vi "LiveAcquire20161118.vi"() -> ()   [LabVIEW 2015]
uses:
  <userlib>/atmcd64d.llb/AcquisitionMode_mode typedef.ctl
  NIDAQControls/StateGlobals.vi
  AcquisitionGlobals.vi
  NIDAQControls/NIDAQGlobals.vi
  LiveImage_Global.vi
panel:
  out "overflow?":bool
  out "deltat":u64
  out "arr":u64[](array[numeric])
  out "size(s) 2":i32
  out "size(s)":i32
  out "xpixels 2":i32
  out "ypixels 2":i32
  out "Acquire Time":dbl
  out "Wait Time":dbl
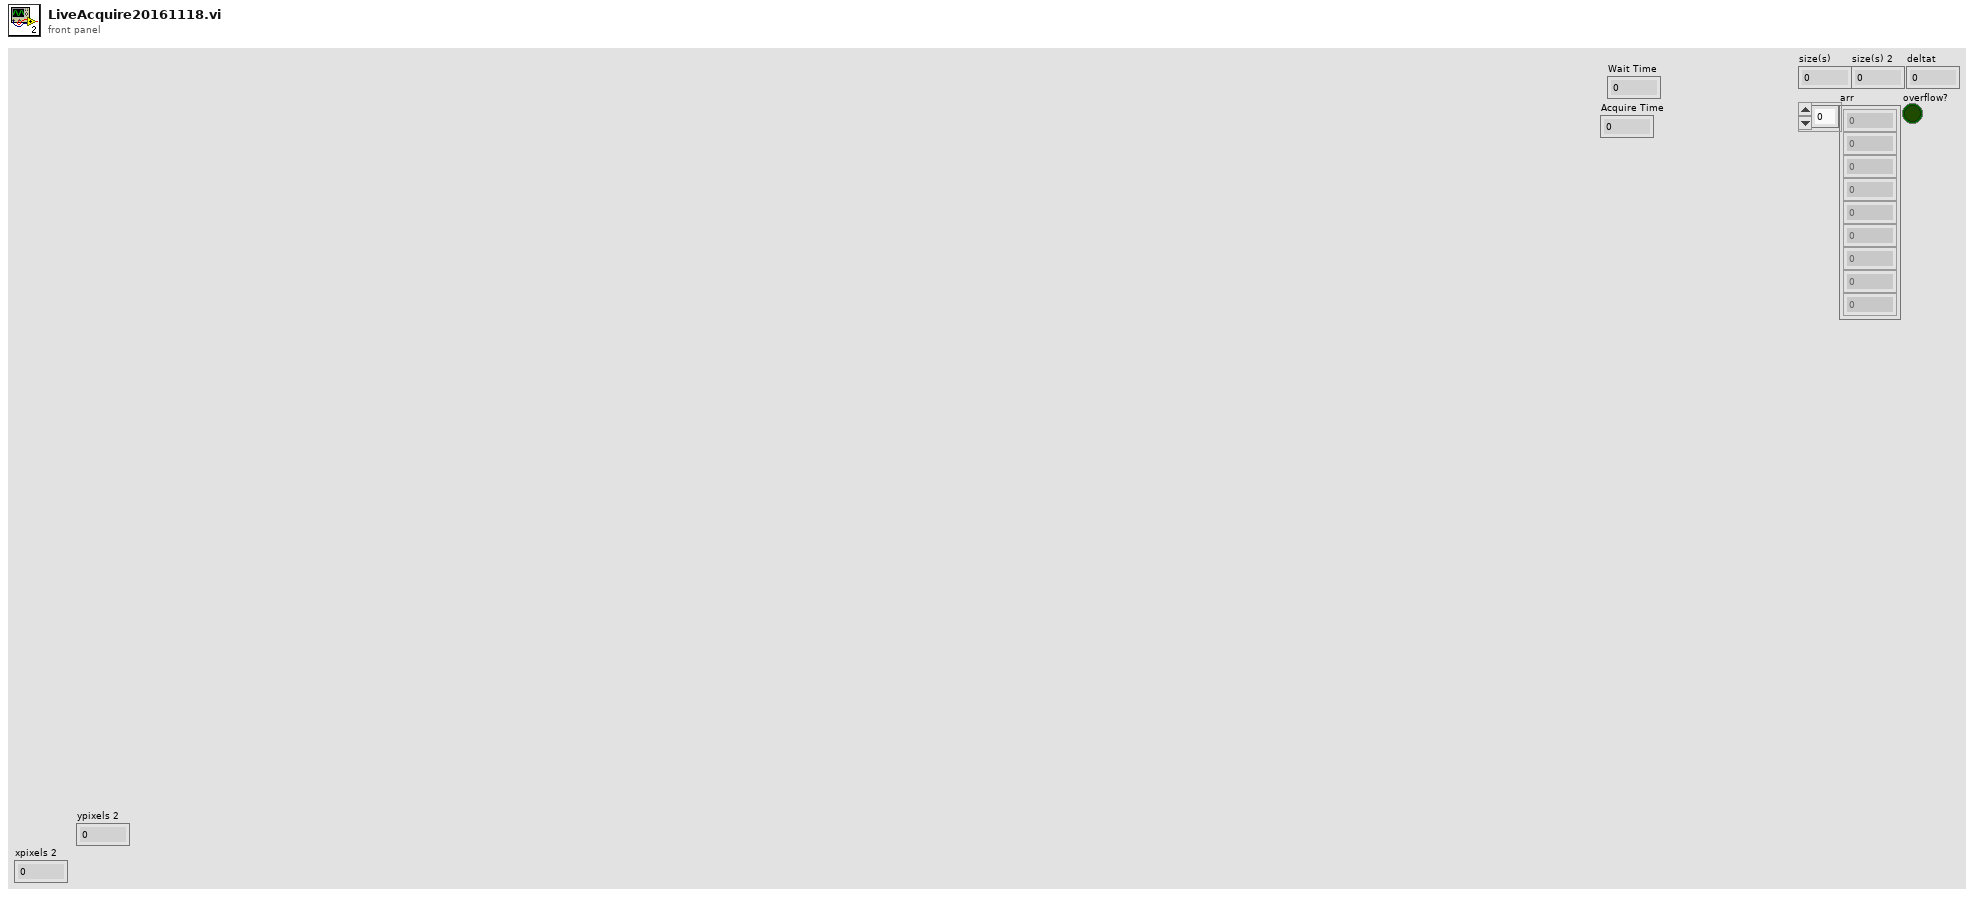
[diagram p1: front panel]
types:
  T1 = cluster{"Start or New Parameters?":bool, "Laser Mode":string, "Piezo Mode":string, "Begin Or End Acquisition":string, "Acquisition Time":dbl}
  T2 = enum16{"Create", "Lossy Enqueue", "Enqueue", "Dequeue", "Destroy"}
  T3 = typedef "AcquisitionMode_mode typedef.ctl" = enum16{"Reserved (0)", "Single Scan", "Accumulate", "Kinetics", "Fast Kinetics", "Run Till Abort", "Reserved (6)", "Reserved (7)", "Reserved (8)", "Time Delayed Integration"}
  T4 = typedef "Rendezvous RefNum" = refnum<k1>
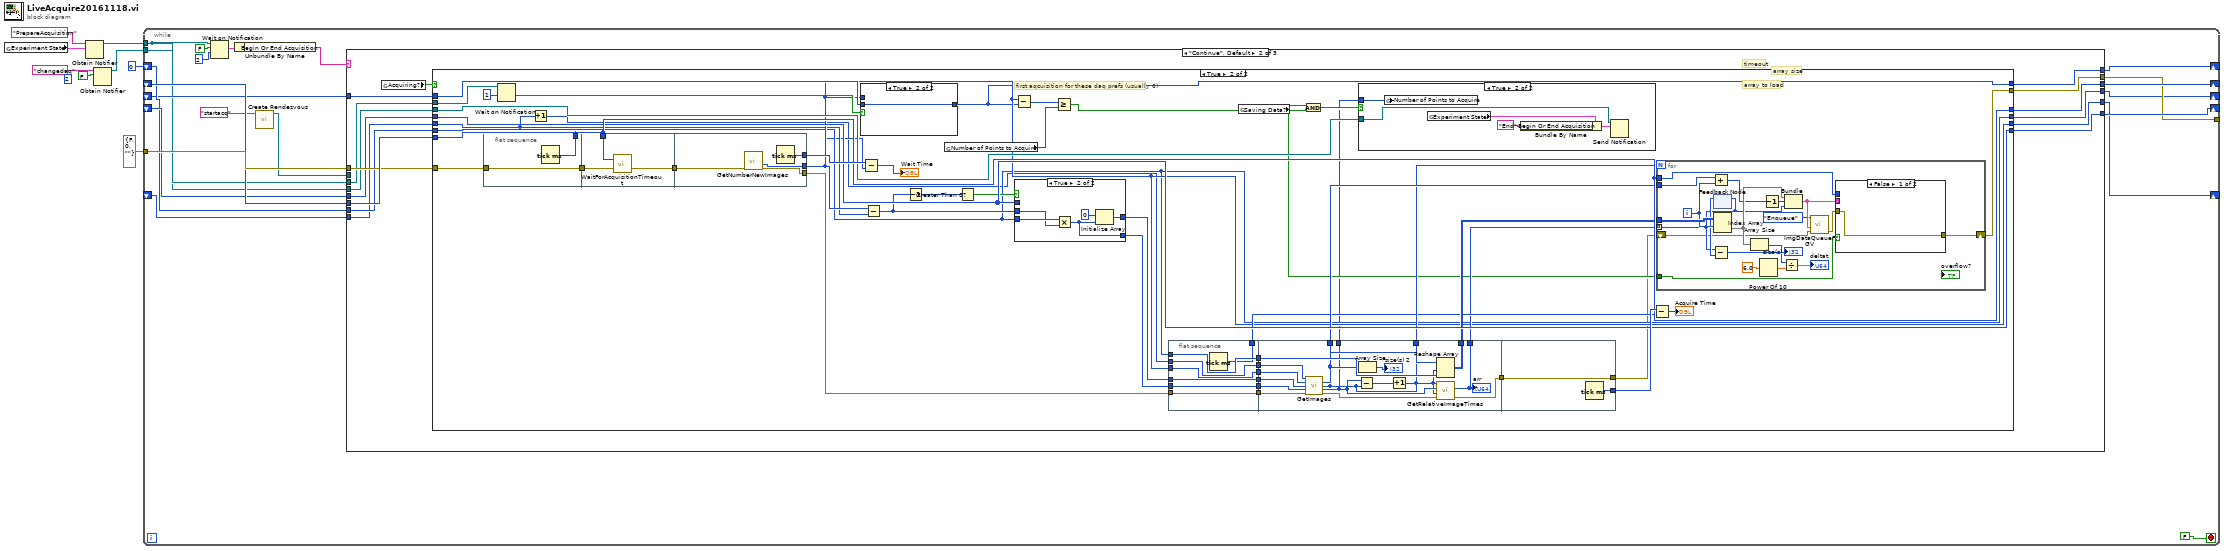
[diagram p0: block diagram]
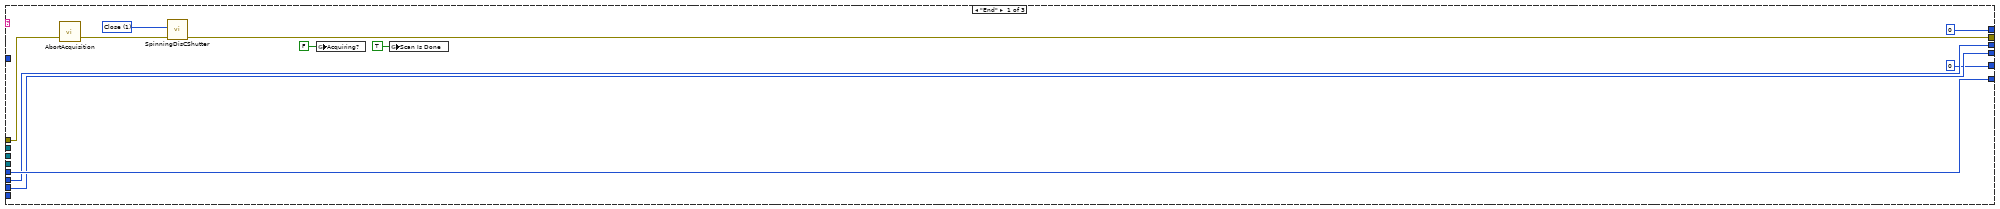
[diagram p2: hidden frame]
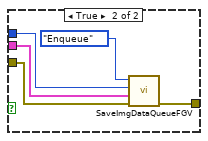
[diagram p4: hidden frame]
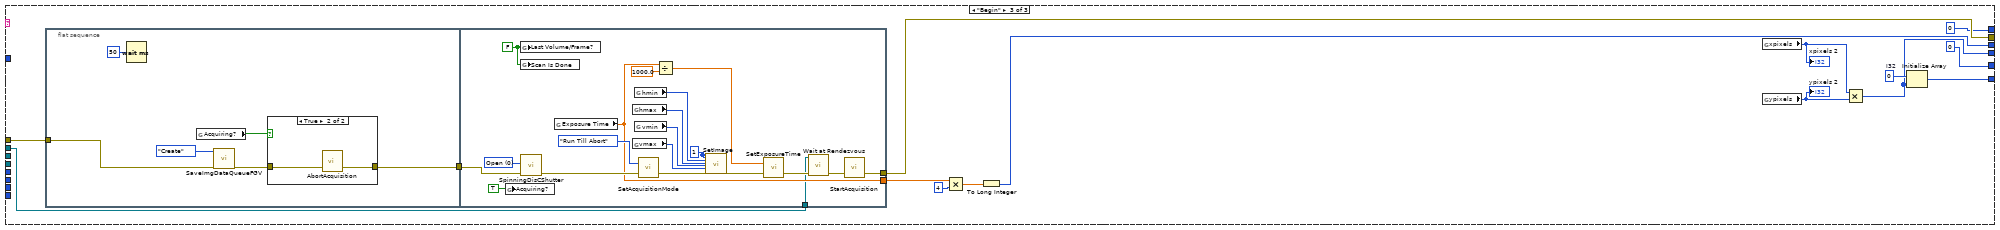
[diagram p8: hidden frame]
diagram:
  (unwired) 2 ("max queue size (-1, unlimited)")
  n1 = global read "StateGlobals.vi" "Experiment State"() -> (w1:T1)
  n2 = Obtain Notifier(name (unnamed)="PrepareAcquisition", notification data type=w1) -> (notifier out=w6:refnum<notifier>)  [unwired: 2 in, 2 out]
  n3 = Obtain Notifier(name (unnamed)="changedaq", notification data type=FALSE) -> (notifier out=w2:refnum<notifier>)  [unwired: 2 in, 2 out]
  n4 = while {
    tunnel: w6 -> [w12]
    shift-right: [w26] -> _
    shift-left: _ -> [w22]
    shift-right: [w25] -> _
    shift-left: _ -> [w21]
    shift-right: [w11] -> _
    shift-left: _ -> [w19]
    tunnel: errorcluster {"status"=FALSE, "code"=0, "source"=""} ("error out") -> [w24]
    tunnel: [w23] -> _
    shift-right: [w14] -> _
    shift-left: 0 -> [w15]
    tunnel: w2 -> [w13]
    shift-right: [w9] -> _
    shift-left: _ -> [w10]
    stop <- FALSE stop-if-true
    # "array size"
    # "timeout"
    # "array to load"
    n5 = Wait on Notification(notifier=w12, ignore previous (F)=FALSE, timeout in ms (-1)=2) -> (notification=w28:T1)  [unwired: 1 in, 3 out]
    n6 = Unbundle By Name(w28) -> ("Begin Or End Acquisition"=w27:string)
    n7 = call <vilib>:"Create Rendezvous.vi"("name (unnamed)"="startacq") -> ("rendezvous"=w17:T4)  [unwired: 4 in, 2 out]
    n8 = case shown="\"Continue\", Default" w27 {
      tunnel: [w33 w48 w191] -> w26
      tunnel: [w35 w49 w190] -> w25
      tunnel: [w34 w47 w189] -> w11
      tunnel: w24 -> [w36 w53 w188]
      tunnel: [w30 w50 w187] -> w23
      tunnel: w22 -> [w33 w54 _]
      tunnel: w21 -> [w35 w52 _]
      tunnel: w19 -> [w34 w51 _]
      tunnel: w17 -> [_ _ w184]
      tunnel: w15 -> [_ w46 _]
      tunnel: [0 ("last") w44 0 ("last")] -> w14
      tunnel: w13 -> [_ w45 _]
      tunnel: w12 -> [_ w43 _]
      tunnel: w10 -> [_ w42 _]
      tunnel: [0 ("last") w41 0 ("last")] -> w9
      frame "End" {
        w38 = u16 1 items=["Open", "Close"] ("Ring")
        n9 = call <userlib>:"AbortAcquisition.vi"("error in (no error)"=w36) -> ("error out"=w37:errorcluster)  [unwired: 1 in, 1 out]
        n10 = call "SpinningDisCShutter.vi"("error in (no error)"=w37, "Ring"=w38) -> ("error out"=w30:errorcluster)  [unwired: 9 in]
        n11 = global write "AcquisitionGlobals.vi" "Acquiring?"(FALSE) -> ()
        n12 = global write "NIDAQGlobals.vi" "Scan Is Done"(TRUE ("Last Volume/Frame?")) -> ()
      }
      frame "Continue", Default {
        n13 = global read "AcquisitionGlobals.vi" "Acquiring?"() -> (w55:bool)
        n14 = case shown="True" w55 {
          tunnel: w54 -> [w58 w98]
          tunnel: w53 -> [w60 w105]
          tunnel: w52 -> [w59 w88]
          tunnel: w51 -> [w61 w69]
          tunnel: [w60 w67] -> w50
          tunnel: [w59 w88] -> w49
          tunnel: [w58 w98] -> w48
          tunnel: [w61 w69] -> w47
          tunnel: w46 -> [w57 w95]
          tunnel: [w57 w62] -> w44
          tunnel: w45 -> [_ w97]
          tunnel: w43 -> [_ w91]
          tunnel: w42 -> [w56 w65]
          tunnel: [w56 w70] -> w41
          frame False {
          }
          frame True {
            # "first aqcuisition for these daq prefs (usually 0)"
            n15 = flat-sequence {
              tunnel: w105 -> [w174]
              tunnel: [w174] -> w107
              tunnel: [w173] -> w64
              tunnel: w107 -> [w177]
              tunnel: [w176] -> w106
              tunnel: w98 -> [w175]
              tunnel: [w179] -> w103
              tunnel: w106 -> [w180]
              tunnel: [w181] -> w101
              tunnel: [w178] -> w70
              frame #0 {
                n16 = Tick Count (ms)() -> (millisecond timer value=w173:u32)
              }
              frame #1 {
                n17 = call <userlib>:"WaitForAcquisitionTimeout.vi"("error in (no error)"=w177, "iTimeOutMs"=w175) -> ("error out"=w176:errorcluster)  [unwired: 1 out]
              }
              frame #2 {
                n18 = call <userlib>:"GetNumberNewImages.vi"("error in (no error)"=w180) -> ("error out"=w179:errorcluster, "last"=w178:i32)  [unwired: 3 in, 2 out]
                n19 = Tick Count (ms)() -> (millisecond timer value=w181:u32)
              }
            }
            n20 = Wait on Notification(notifier=w97, timeout in ms (-1)=1) -> (timed out?=w96:bool)  [unwired: 2 in, 3 out]
            n21 = Increment(x=w65) -> (x+1=w63:i32)
            n22 = case shown="True" w96 {
              tunnel: w95 -> [_ w147]
              tunnel: w70 -> [w146 _]
              tunnel: [w146 w147] -> w62
              frame False {
              }
              frame True {
              }
            }
            n23 = Subtract(x=w101, y=w64) -> (x-y=→"Wait Time":u32)
            n24 = Subtract(x=w70, y=w65) -> (x-y=w84:i32)
            n25 = Decrement(x=w84) -> (x-1=w81:i32)
            n26 = global read "StateGlobals.vi" "Number of Points to Acquire"() -> (w93:i32)
            n27 = Greater Than 0?(x=w81) -> (x > 0?=w85:bool)
            n28 = case shown="True" w85 {
              tunnel: w69 -> [w134 w139]
              tunnel: w88 -> [w135 _]
              tunnel: [w135 w137] -> w87
              tunnel: [w134 w136] -> w86
              tunnel: w84 -> [_ w138]
              frame False {
              }
              frame True {
                n29 = Multiply(x=w139, y=w138) -> (x*y=w136:i32)
                n30 = Initialize Array(u16 0 ("element"), w136) -> (w137:u16[])
              }
            }
            n31 = Subtract(x=w70, y=w62) -> (x-y=w89:i32)
            n32 = Greater Or Equal?(x=w89, y=w93) -> (x >= y?=w92:bool)
            n33 = flat-sequence {
              tunnel: w69 -> [w149]
              tunnel: w86 -> [w150]
              tunnel: w63 -> [w151]
              tunnel: w70 -> [w152]
              tunnel: w103 -> [w153]
              tunnel: w87 -> [w154]
              tunnel: [w154] -> w79
              tunnel: [w153] -> w78
              tunnel: [w152] -> w77
              tunnel: [w151] -> w76
              tunnel: [w150] -> w75
              tunnel: [w149] -> w74
              tunnel: [w148] -> w73
              tunnel: [w161] -> w104
              tunnel: [w166] -> w83
              tunnel: [w160] -> w82
              tunnel: [w155] -> w80
              tunnel: w79 -> [w168]
              tunnel: w78 -> [w170]
              tunnel: w77 -> [w169]
              tunnel: w76 -> [w156]
              tunnel: w75 -> [w167]
              tunnel: w74 -> [w165]
              tunnel: [w158] -> w72
              tunnel: [w157] -> w66
              tunnel: [w172] -> w68
              tunnel: w104 -> [w172]
              tunnel: [w171] -> w100
              frame #0 {
                n34 = Tick Count (ms)() -> (millisecond timer value=w148:u32)
              }
              frame #1 {
                n35 = call <userlib>:"GetImages.vi"("first"=w156, "last"=w169, "array"=w168, "size"=w167, "error in (no error)"=w170) -> ("array"=w164:i32[], "validfirst"=w160:i32, "validlast"=w157:i32, "error out"=w162:errorcluster)  [unwired: 6 in, 1 out]
                n36 = Subtract(x=w157, y=w160) -> (x-y=w159:i32)
                n37 = Array Size(array=w164) -> (size(s)=→"size(s) 2":i32)
                n38 = Increment(x=w159) -> (x+1=w155:i32)
                n39 = Reshape Array(w164, w155, w165) -> (w166:i32[][])
                n40 = call <userlib>:"GetRelativeImageTimes.vi"("error in (no error)"=w162, "size"=w155, "last"=w157, "first"=w160) -> ("error out"=w161:errorcluster, "arr"=w158:u64[])  [unwired: 5 in, 1 out]
                "arr" <- w158
              }
              frame #2 {
                n41 = Tick Count (ms)() -> (millisecond timer value=w171:u32)
              }
            }
            n42 = global read "AcquisitionGlobals.vi" "Saving Data?"() -> (w71:bool)
            n43 = And(x=w71, y=w92) -> (x .and. y?=w90:bool)
            n44 = case shown="True" w90 {
              tunnel: w91 -> [_ w145]
              tunnel: w66 -> [_ w141]
              frame False {
              }
              frame True {
                n45 = global write "StateGlobals.vi" "Number of Points to Acquire"(w141) -> ()
                n46 = global read "StateGlobals.vi" "Experiment State"() -> (w144:T1)
                n47 = Bundle By Name(cluster=w144, "Begin Or End Acquisition"="End") -> (w142:T1)
                n48 = Send Notification(notification=w142, notifier=w145) -> ()  [unwired: 1 in, 2 out]
              }
            }
            n49 = Subtract(x=w100, y=w73) -> (x-y=→"Acquire Time":u32)
            n50 = for {
              N: w80 -> [_]
              tunnel: w98 -> [w127]
              tunnel: w71 -> [w115]
              tunnel: w83 -> [w124]
              tunnel: w82 -> [w126]
              tunnel: w72 -> [w120] mode=indexing
              shift-right: [w110] -> w67
              shift-left: w68 -> [w112]
              i -> [w122]
              n51 = Add(x=w126, y=w122) -> (x+y=w109:i32)
              n52 = feedback-in #1(w120) -> ()
              n53 = feedback #1() -> (w121:u64)  [unwired: 1 in]
              n54 = Subtract(x=w120, y=w121) -> (x-y=w119:u64)
              n55 = Index Array(array=w124, index (row)=w122) -> (element=w123:i32[])  [unwired: 1 in]
              n56 = Array Size(array=w123) -> (size(s)=→"size(s)":i32)
              n57 = Power Of 10(x=6.0) -> (10^x=w116:dbl)
              n58 = Decrement(x=w109) -> (x-1=w108:i32)
              n59 = Divide(x=w119, y=w116) -> (x/y=→"deltat":dbl)
              n60 = Bundle("array"=w123, w108, w120) -> (w114:cluster{"array":i32[], i32, u64})  [unwired: 1 in]
              n61 = call "ImgDataQueueFGV.vi"("error out"=w112, "Data In"=w114, "Action"=T2."Enqueue") -> ("error out 2"=w111:errorcluster)  [unwired: 6 in, 2 out]
              n62 = case shown="False" w115 {
                tunnel: w127 -> [_ w129]
                tunnel: w114 -> [_ w133]
                tunnel: w111 -> [w128 w132]
                tunnel: [w128 w131] -> w110
                frame False {
                }
                frame True {
                  n63 = call "SaveImgDataQueueFGV.vi"("error out"=w132, "Data In"=w133, "timeout in ms (-1)"=w129, "Action"=T2."Enqueue") -> ("error out 2"=w131:errorcluster)  [unwired: 5 in, 2 out]
                }
              }
            }
          }
        }
      }
      frame "Begin" {
        w194 = u16 0  # I32
        n64 = flat-sequence {
          tunnel: w188 -> [w199]
          tunnel: [w202] -> w186
          tunnel: [w221] -> w187
          tunnel: w186 -> [w222]
          tunnel: [w209] -> w185
          tunnel: w184 -> [w206]
          frame #0 {
            n65 = Wait (ms)(milliseconds to wait=u32 50) -> ()  [unwired: 1 out]
            n66 = global read "AcquisitionGlobals.vi" "Acquiring?"() -> (w201:bool)
            n67 = call "SaveImgDataQueueFGV.vi"("error out"=w199, "Action"=T2."Create") -> ("error out 2"=w198:errorcluster)  [unwired: 7 in, 2 out]
            n68 = case shown="True" w201 {
              tunnel: w198 -> [w203 w205]
              tunnel: [w203 w204] -> w202
              frame False {
              }
              frame True {
                n69 = call <userlib>:"AbortAcquisition.vi"("error in (no error)"=w205) -> ("error out"=w204:errorcluster)  [unwired: 1 in, 1 out]
              }
            }
          }
          frame #1 {
            w218 = 1
            w220 = FALSE ("Last Volume/Frame?")
            w224 = u16 0 items=["Open", "Close"] ("Ring")
            n70 = global write "AcquisitionGlobals.vi" "Acquiring?"(TRUE) -> ()
            n71 = global write "NIDAQGlobals.vi" "Last Volume/Frame?"(w220) -> ()
            n72 = global write "NIDAQGlobals.vi" "Scan Is Done"(w220) -> ()
            n73 = call "SpinningDisCShutter.vi"("error in (no error)"=w222, "Ring"=w224) -> ("error out"=w223:errorcluster)  [unwired: 9 in]
            n74 = global read "LiveImage_Global.vi" "Exposure Time"() -> (w209:dbl)
            n75 = global read "LiveImage_Global.vi" "hmax"() -> (w216:i32)
            n76 = global read "LiveImage_Global.vi" "vmax"() -> (w214:i32)
            n77 = global read "LiveImage_Global.vi" "hmin"() -> (w217:i32)
            n78 = global read "LiveImage_Global.vi" "vmin"() -> (w215:i32)
            n79 = call <userlib>:"SetAcquisitionMode.vi"("error in (no error)"=w223, "mode"=AcquisitionMode_mode_typedef."Run Till Abort") -> ("error out"=w213:errorcluster)  [unwired: 1 out]
            n80 = Divide(x=w209, y=1000.0) -> (x/y=w210:dbl)
            n81 = call <userlib>:"SetImage.vi"("hbin"=w218, "vbin"=w218, "hstart"=w217, "hend"=w216, "vstart"=w215, "vend"=w214, "error in (no error)"=w213) -> ("error out"=w212:errorcluster)  [unwired: 19 in, 1 out]
            n82 = call <userlib>:"SetExposureTime.vi"("error in (no error)"=w212, "time"=w210) -> ("error out"=w208:errorcluster)  [unwired: 1 out]
            n83 = call <vilib>:"Wait at Rendezvous.vi"("error in (no error)"=w208, "rendezvous"=w206) -> ("error out"=w207:errorcluster)  [unwired: 3 in, 2 out]
            n84 = call <userlib>:"StartAcquisition.vi"("error in (no error)"=w207) -> ("error out"=w221:errorcluster)  [unwired: 1 in, 1 out]
          }
        }
        n85 = Multiply(x=w185, y=4) -> (x*y=w192:dbl)
        n86 = To Long Integer(number=w192) -> (32bit integer=w191:i32)
        n87 = global read "LiveImage_Global.vi" "xpixels"() -> (w195:i32)
        "xpixels 2" <- w195
        n88 = global read "LiveImage_Global.vi" "ypixels"() -> (w196:i32)
        "ypixels 2" <- w196
        n89 = Multiply(x=w195, y=w196) -> (x*y=w189:i32)
        n90 = Initialize Array "Initialize Array"(w194, w189) -> (w190:u16[])
      }
    }
  }
